vi "Open Hardware.vi"(8 "error in (no error)":errorcluster, 11 "Inst.Attocube-3DR in":refnum<class "Inst.Attocube-3DR.lvclass">) -> (0 "error out":errorcluster, 3 "Inst.Attocube-3DR out":refnum<class "Inst.Attocube-3DR.lvclass">)   [LabVIEW 2019, in "Inst.Attocube-3DR.lvclass"]
uses:
  Inst.Attocube-3DR.lvclass
  Inst.Attocube-3DR.lvclass/Inst.Attocube-3DR.ctl
  <userlib>/LevyLab/Instrument Framework/Instrument Types/VSource/Instrument.VSource.lvclass
  <userlib>/LevyLab/Instrument Framework/SMOs/Instrument/Instrument.lvclass
  C:/Program Files (x86)/National Instruments/LabVIEW 2019/user.lib/LevyLab/Instrument Framework/SMOs/Instrument/Instrument.lvclass
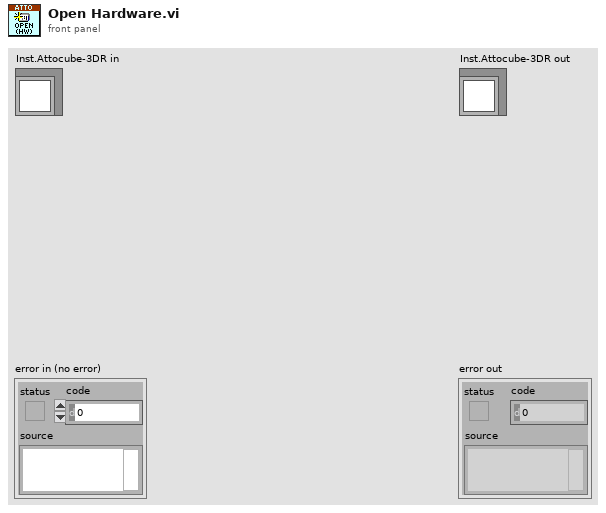
[diagram p1: front panel]
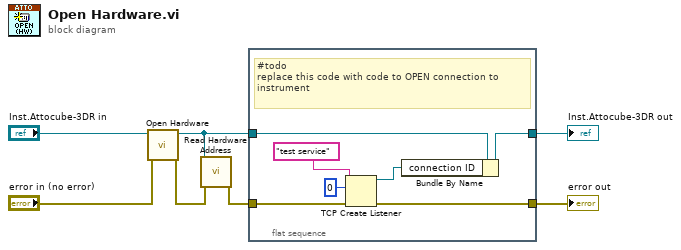
[diagram p0: block diagram]
diagram:
  n1 = call-parent "Open Hardware.vi"("error in (no error)"="error in (no error)", "Instrument in"="Inst.Attocube-3DR in") -> ("error out"=w5:errorcluster, "Instrument out"=w4:refnum<class "Inst.Attocube-3DR.lvclass">)  [unwired: 8 in]
  n2 = call <userlib>:"Read Hardware Address.vi"("error in (no error)"=w5, "Instrument in"=w4) -> ("error out"=w2:errorcluster)  [unwired: 7 in, 2 out]
  n3 = flat-sequence {
    tunnel: w4 -> [w14]
    tunnel: [w13] -> w3
    tunnel: w2 -> [w12]
    tunnel: [w11] -> w1
    frame #0 {
      # "#todo\nreplace this code with code to OPEN connection to instrument"
      n4 = TCP Create Listener(8:w12, 10:u16 0 ("port"), 11:"test service" ("service name")) -> (0:w11:errorcluster, 3:w9:refnum<k5>)  [unwired: 2 in, 1 out]
      n5 = Bundle By Name(cluster=w14, "connection ID"=w9) -> (w13:refnum<class "Inst.Attocube-3DR.lvclass">)
    }
  }
  "error out" <- w1
  "Inst.Attocube-3DR out" <- w3
